vi "Toggle.vi"(10 "FlashInput":bool) -> (2 "On/Off":bool)   [LabVIEW 2020]
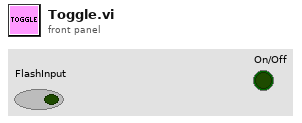
[diagram p1: front panel]
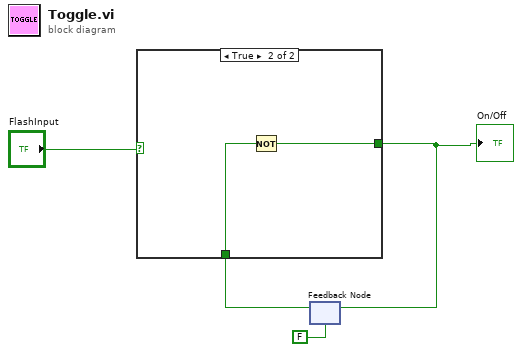
[diagram p0: block diagram]
diagram:
  n1 = feedback #1(FALSE) -> (w3:bool)
  n2 = case shown="True" "FlashInput" {
    tunnel: w3 -> [w5 w7]
    tunnel: [w5 w6] -> w1
    frame False {
    }
    frame True {
      n3 = Not(x=w7) -> (.not. x?=w6:bool)
    }
  }
  "On/Off" <- w1
  n4 = feedback-in #1(w1) -> ()
